vi "PH_TKTDS-30xx.Evt Call Set Channel Position.vi"(0 "i ref in":refnum<vi>, 1 "Instance":string="N/A", 2 "Channel to be positioned":string(combo)="CH1", 3 "Position":dbl, 5 "error in (no error)":errorcluster) -> (14 "i ref out":refnum<vi>, 19 "error out":errorcluster)   [LabVIEW 2014, in "PH_TKTDS-30xx.lvlib"]
doc: "This VI calls sets a simple call."
uses:
  PH_TKTDS-30xx.lvlib
  CS_Core/CSSystem/CoreLib/CoreLib.double 2 byte array.vi
  CS_Core/CSSystem/CoreLib/CoreLib.string 2 byte array.vi
  CS_Core/CSSystem/CoreLib/CoreLib.lvlib
  CS_Core/BaseProcess/BaseProcess.lvlib
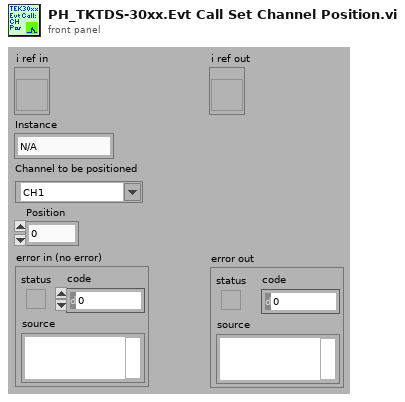
[diagram p1: front panel]
types:
  T1 = typedef "CoreDefs.rawDataType.ctl" = i8[]
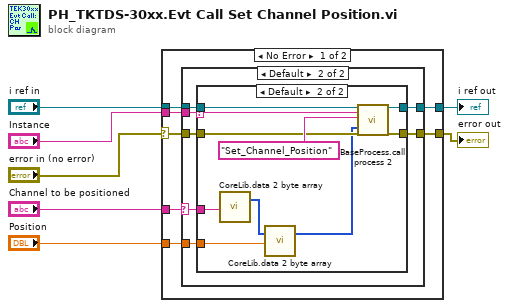
[diagram p0: block diagram]
diagram:
  n1 = case shown="No Error" "error in (no error)" {
    selector: "error in (no error)" -> [w10 w36]
    tunnel: [w14 w37] -> w7
    tunnel: [w13 w36] -> w6
    tunnel: "i ref in" -> [w12 w37]
    tunnel: "Channel to be positioned" -> [w9 _]
    tunnel: "Instance" -> [w11 _]
    tunnel: "Position" -> [w8 _]
    frame No Error {
      n2 = case shown="Default" w9 {
        selector: w9 -> [_ w18]
        tunnel: [w16 w23] -> w14
        tunnel: [w15 w22] -> w13
        tunnel: w12 -> [w16 w21]
        tunnel: w11 -> [_ w20]
        tunnel: w10 -> [w15 w19]
        tunnel: w8 -> [_ w17]
        frame "", "N/A" {
        }
        frame Default {
          n3 = case shown="Default" w20 {
            selector: w20 -> [_ w30]
            tunnel: [w24 w34] -> w23
            tunnel: [w25 w33] -> w22
            tunnel: w21 -> [w24 w32]
            tunnel: w19 -> [w25 w31]
            tunnel: w18 -> [_ w29]
            tunnel: w17 -> [_ w28]
            frame "N/A" {
            }
            frame Default {
              n4 = call-poly "CoreLib.data 2 byte array.vi"("string"=w29) -> ("byteArray out"=w26:T1)  [unwired: 18 in]
              n5 = call-poly "CoreLib.data 2 byte array.vi"("byteArray"=w26, "f64"=w28) -> ("byteArray out"=w27:T1)  [unwired: 17 in]
              n6 = call "BaseProcess.call process 2.vi"("i ref in"=w32, "Object"=w30, "Selector"="Set_Channel_Position", "Data"=w27, "error in (no error)"=w31) -> ("i ref out"=w34:refnum<vi>, "error out"=w33:errorcluster)  [unwired: 13 in]
            }
          }
        }
      }
    }
    frame Error {
    }
  }
  "i ref out" <- w7
  "error out" <- w6
